vi "JoystickToBool (SubVI).vi"(10 "Treshhold":dbl, 11 "Axis":dbl) -> (2 "AutoForward":bool, 3 "AutoTurn":bool)   [LabVIEW 2018, in "Joysticks.lvlib" / "Two Drivers.lvclass"]
uses:
  Two Drivers.lvclass
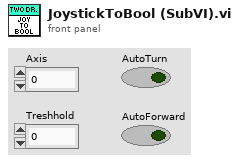
[diagram p1: front panel]
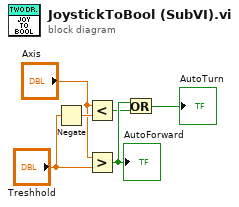
[diagram p0: block diagram]
diagram:
  n1 = Negate(x="Treshhold") -> (-x=w2:dbl)
  n2 = Less?(x="Axis", y=w2) -> (x < y?=w4:bool)
  n3 = Greater?(x="Axis", y="Treshhold") -> (0:w6:bool)
  "AutoForward" <- w6
  n4 = Or(x=w6, y=w4) -> (x .or. y?=→"AutoTurn":bool)
